vi "Get Channel Table.vi"(8 "error in (no error)":errorcluster, 10 "Instrument Model (54621D)":string="54621D", 11 "VISA Resource Name":refnum<visa-resource-name>) -> (0 "error out":errorcluster, 2 "Channel Table":string[](array[string]), 3 "VISA Resource Name Out":refnum<visa-resource-name>)   [LabVIEW 2011, in "Agilent 546XX Series.lvlib"]
doc: "Returns the correct array list of channels that the current instrument model supports."
uses:
  Agilent 546XX Series.lvlib
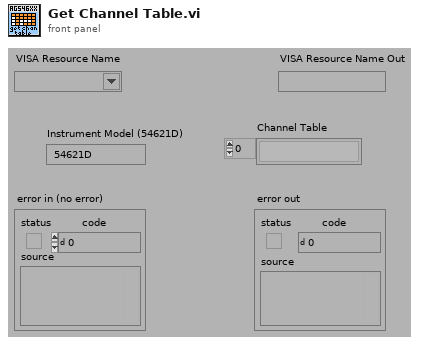
[diagram p1: front panel]
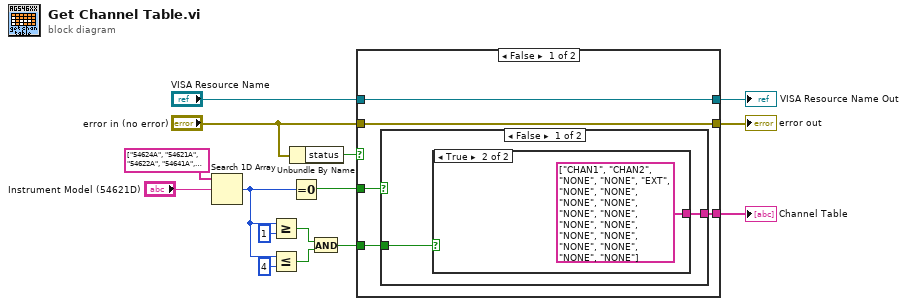
[diagram p0: block diagram]
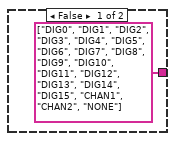
[diagram p2: hidden frame]
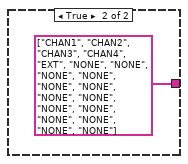
[diagram p3: hidden frame]
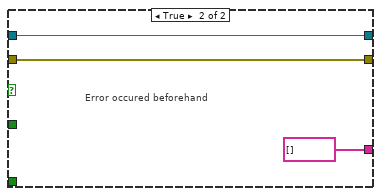
[diagram p4: hidden frame]
diagram:
  n1 = Search 1D Array(1D array=string[] ["54624A", "54621A", "54622A", "54641A", "54642A", "54621D", "54622D", "54641D", "54642D"], element="Instrument Model (54621D)") -> (index of element=w5:i32)  [unwired: 1 in]
  n2 = Greater Or Equal?(x=w5, y=1) -> (x >= y?=w7:bool)
  n3 = Less Or Equal?(x=w5, y=4) -> (x <= y?=w6:bool)
  n4 = Unbundle By Name("error in (no error)") -> ("status"=w15:bool)
  n5 = Equal To 0?(x=w5) -> (x = 0?=w8:bool)
  n6 = And(x=w7, y=w6) -> (x .and. y?=w2:bool)
  n7 = case shown="False" w15 {
    tunnel: "error in (no error)" -> [w19 w27]
    tunnel: "VISA Resource Name" -> [w20 w28]
    tunnel: [w20 w28] -> w12
    tunnel: [w19 w27] -> w11
    tunnel: w8 -> [w18 _]
    tunnel: w2 -> [w17 _]
    tunnel: [w16 string[] []] -> w1
    frame False {
      n8 = case shown="False" w18 {
        tunnel: w17 -> [w22 _]
        tunnel: [w21 string[] ["CHAN1", "CHAN2", "CHAN3", "CHAN4", "EXT", "NONE", "NONE", "NONE", "NONE", "NONE", "NONE", "NONE", "NONE", "NONE", "NONE", "NONE", "NONE", "NONE", "NONE"]] -> w16
        frame False {
          n9 = case shown="True" w22 {
            tunnel: [string[] ["DIG0", "DIG1", "DIG2", "DIG3", "DIG4", "DIG5", "DIG6", "DIG7", "DIG8", "DIG9", "DIG10", "DIG11", "DIG12", "DIG13", "DIG14", "DIG15", "CHAN1", "CHAN2", "NONE"] string[] ["CHAN1", "CHAN2", "NONE", "NONE", "EXT", "NONE", "NONE", "NONE", "NONE", "NONE", "NONE", "NONE", "NONE", "NONE", "NONE", "NONE", "NONE", "NONE", "NONE"]] -> w21
            frame False {
            }
            frame True {
            }
          }
        }
        frame True {
        }
      }
    }
    frame True {
      # "Error occured beforehand"
    }
  }
  "VISA Resource Name Out" <- w12
  "error out" <- w11
  "Channel Table" <- w1
